vi "Send.vi"(8 "error in":errorcluster, 11 "SDO Transfer in":refnum<class "SDO Transfer.lvclass">) -> (0 "error out":errorcluster, 3 "SDO Transfer out":refnum<class "SDO Transfer.lvclass">)   [LabVIEW 2020, in "CANopen.lvlib" / "SDO Manager.lvlib" / "SDO Transfer.lvclass"]
uses:
  SDO Transfer.lvclass
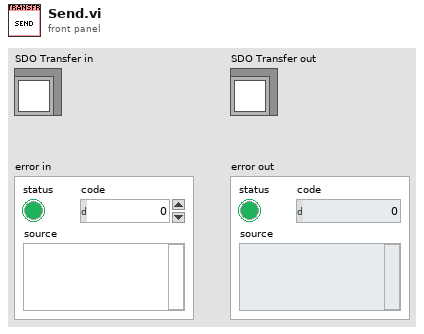
[diagram p1: front panel]
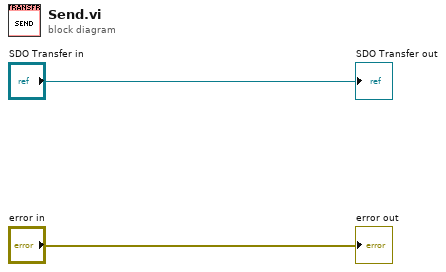
[diagram p0: block diagram]
diagram:
  "SDO Transfer out" <- "SDO Transfer in"
  "error out" <- "error in"
